vi "DialogCreateLib.vi"(0 "LibWriter":refnum<class "LibWriter.lvclass">, 1 "ProjectItem Refnum":refnum<vi>, 5 "error in (no error)":errorcluster) -> (14 "LibWriter":refnum<class "LibWriter.lvclass">, 15 "Cancelled":bool, 16 "CreateLibData":T1, 17 "DesignPatternsToAddAfterCreation":string[](array[string]), 18 "ChangeProviderRequested":string, 19 "error out":errorcluster)   [LabVIEW 2014, in "LibWriter.lvclass"]
uses:
  <resource>/Framework/Providers/Open_GDS/ClassProviders/LibProvider_BaseClassInterface/LibWriter_class/ClassWriter_class/LibWriter.lvclass
  <resource>/Framework/Providers/Open_GDS/ClassProviders/LibProvider_BaseClassInterface/LibWriter_class/CreateLibData.vi
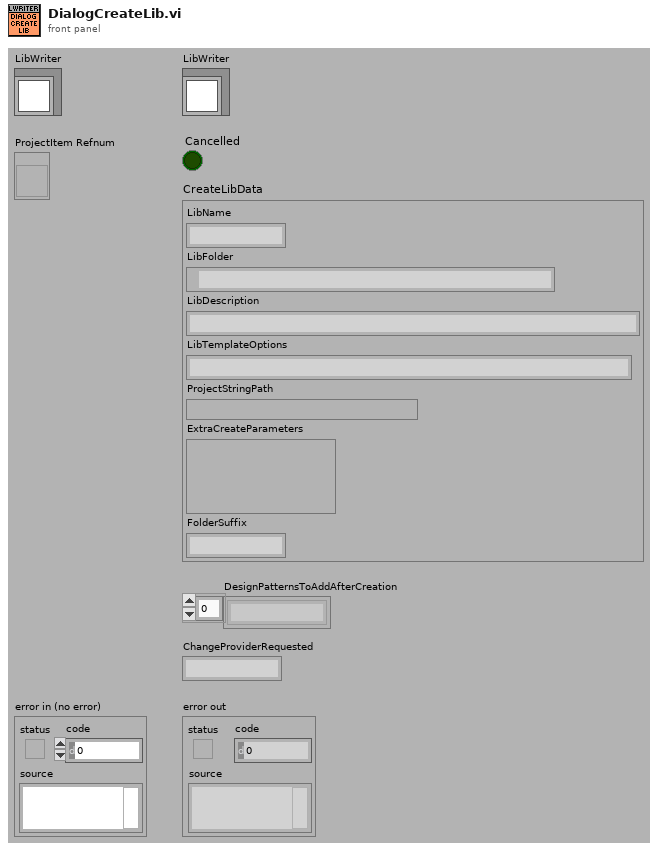
[diagram p1: front panel]
types:
  T1 = typedef "LibWriter.lvclass/CreateLibData.vi" = cluster{"LibName":string, "LibFolder":path, "LibDescription":string, "LibTemplateOptions":string, "ProjectStringPath":variant, "ExtraCreateParameters":variant, "FolderSuffix":string}
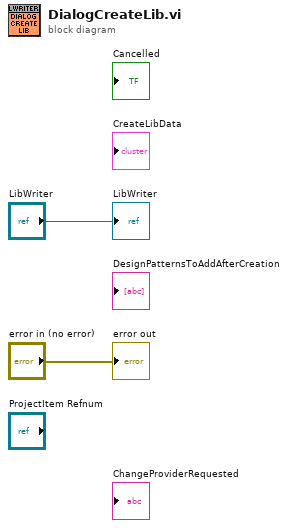
[diagram p0: block diagram]
diagram:
  "error out" <- "error in (no error)"
  "LibWriter" <- "LibWriter"
